vi "CreateSensorSession.vi"(8 "error in (no error)":errorcluster, 11 "SiemensDigitalEnergyMeter in":refnum<class "SiemensDigitalEnergyMeter.lvclass">) -> (0 "error out":errorcluster, 3 "SiemensDigitalEnergyMeter out":refnum<class "SiemensDigitalEnergyMeter.lvclass">)   [LabVIEW 2018, in "SensorPlugins.lvlib" / "SiemensDigitalEnergyMeter.lvclass"]
doc: "This VI opens a communication link between the application and the Siemens Digital Energy Meter using an IP address and a port number."
uses:
  SiemensDigitalEnergyMeter.lvclass
  <vilib>/NI/Modbus Library/API/Wrapper/Create Serial Master.vi
  <vilib>/NI/Modbus Library/API/Wrapper/Create TCP Master.vi
  <vilib>/NI/Modbus Library/API/Master/Modbus Master.lvclass
  <vilib>/NI/Modbus Library/API/Wrapper/API Main.lvlib
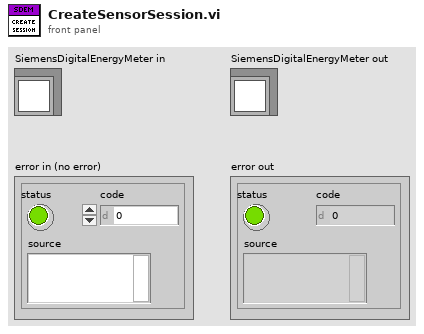
[diagram p1: front panel]
types:
  T1 = typedef "SensorPlugins.lvlib/SiemensDigitalEnergyMeter.lvclass/SiemensDigitalEnergyMeterControls.ctl" = cluster{"Measurement(s)":u16[], "Configuration Commands":string, "Use Measurement Commands Text Box?":bool, "Measurement Commands":string, "Connected?":bool, "Serial Number":string, "IP Address":string, "Port (502)":u16, "Unit ID":u8, "Serial Type":enum16{"RTU", "ASCII"}, "Using TCP?":bool, "VISA Resource Name":string}[]
  T2 = typedef "SensorPlugins.lvlib/SiemensDigitalEnergyMeter.lvclass/CommunicationControls.ctl" = refnum<class "Modbus Master.lvclass">[]
  T3 = cluster{"Measurement(s)":u16[], "Configuration Commands":string, "Use Measurement Commands Text Box?":bool, "Measurement Commands":string, "Connected?":bool, "Serial Number":string, "IP Address":string, "Port (502)":u16, "Unit ID":u8, "Serial Type":enum16{"RTU", "ASCII"}, "Using TCP?":bool, "VISA Resource Name":string}
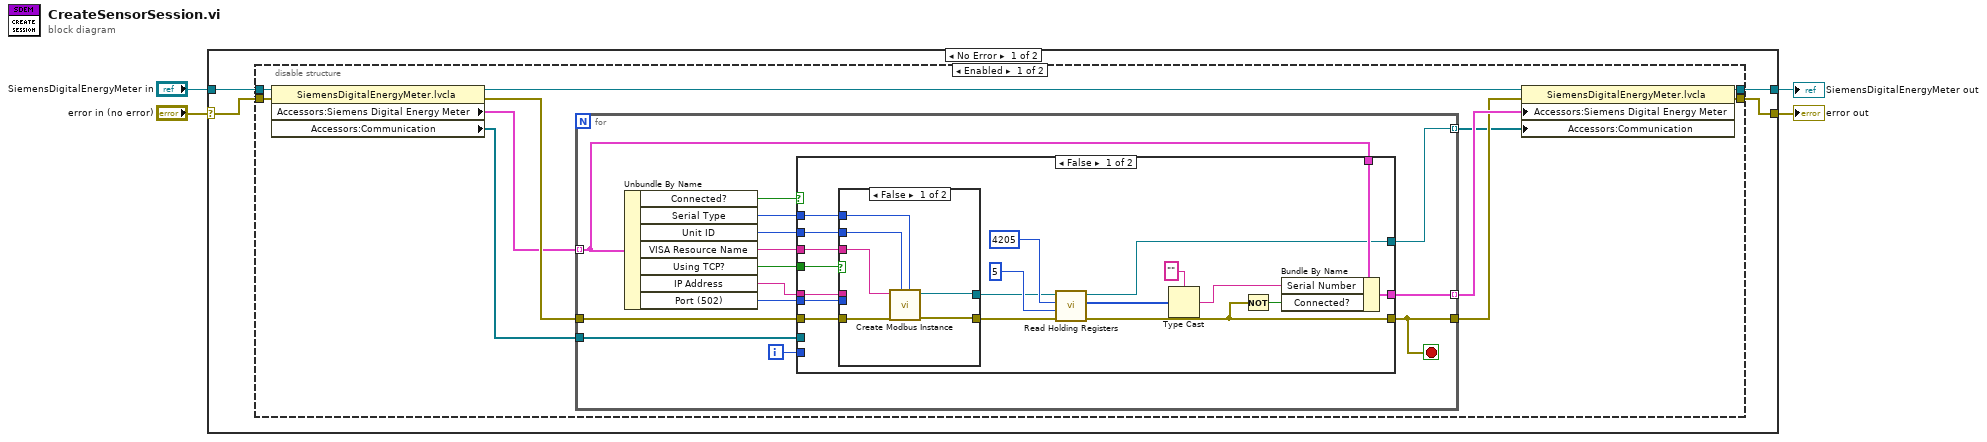
[diagram p0: block diagram]
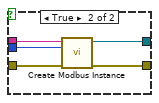
[diagram p2: hidden frame]
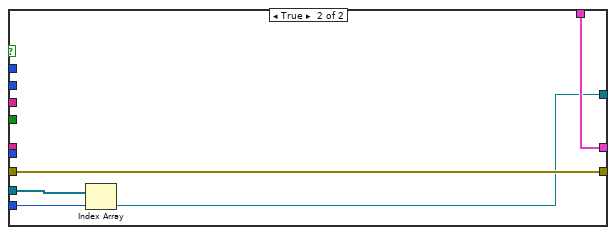
[diagram p3: hidden frame]
diagram:
  n1 = case shown="No Error" "error in (no error)" {
    selector: "error in (no error)" -> [w7 w71]
    tunnel: "SiemensDigitalEnergyMeter in" -> [w8 w72]
    tunnel: [w6 w72] -> w2
    tunnel: [w5 w71] -> w1
    frame No Error {
      n2 = disable-structure shown="Enabled" {
        disable-tunnel: w8 -> [w19 w70]
        disable-tunnel: w7 -> [w18 w69]
        disable-tunnel: [w15 w70] -> w6
        disable-tunnel: [w11 w69] -> w5
        frame Enabled {
          n3 = property class="SiemensDigitalEnergyMeter.lvcla"(reference=w19, error in=w18) -> (reference out=w14:refnum<class "SiemensDigitalEnergyMeter.lvclass">, error out=w17:errorcluster, "Accessors:Siemens Digital Energy Meter"=w16:T1, "Accessors:Communication"=w9:T2)
          n4 = for {
            tunnel: w17 -> [w31]
            tunnel: [w28] -> w12
            tunnel: w16 -> [w33] mode=indexing
            tunnel: [w32] -> w13 mode=indexing
            tunnel: [w27] -> w10 mode=indexing
            tunnel: w9 -> [w20]
            i -> [w21]
            stop <- w28 stop-if-true
            n5 = Unbundle By Name(w33) -> ("Connected?"=w22:bool, "Serial Type"=w23:enum16{"RTU", "ASCII"}, "Unit ID"=w24:u8, "VISA Resource Name"=w25:string, "Using TCP?"=w26:bool, "IP Address"=w30:string, "Port (502)"=w29:u16)
            n6 = case shown="False" w22 {
              tunnel: w33 -> [w52 w68]
              tunnel: [w51 w68] -> w32
              tunnel: w31 -> [w47 w67]
              tunnel: w30 -> [w46 _]
              tunnel: w29 -> [w45 _]
              tunnel: [w44 w67] -> w28
              tunnel: [w38 w64] -> w27
              tunnel: w26 -> [w37 _]
              tunnel: w25 -> [w36 _]
              tunnel: w24 -> [w35 _]
              tunnel: w23 -> [w34 _]
              tunnel: w21 -> [_ w66]
              tunnel: w20 -> [_ w65]
              frame False {
                n7 = case shown="False" w37 {
                  tunnel: w47 -> [w58 w63]
                  tunnel: w46 -> [_ w62]
                  tunnel: w45 -> [_ w61]
                  tunnel: [w57 w60] -> w43
                  tunnel: [w56 w59] -> w40
                  tunnel: w36 -> [w55 _]
                  tunnel: w35 -> [w54 _]
                  tunnel: w34 -> [w53 _]
                  frame False {
                    n8 = call-poly <vilib>:"Create Modbus Instance.vi"("serial type"=w53, "unit ID"=w54, "error in"=w58, "VISA resource name"=w55) -> ("error out"=w57:errorcluster, "serial master instance"=w56:refnum<class "Modbus Master.lvclass">)  [unwired: 6 in]
                  }
                  frame True {
                    n9 = call-poly <vilib>:"Create Modbus Instance.vi"("error in"=w63, "port (502)"=w61, "address"=w62) -> ("error out"=w60:errorcluster, "TCP master instance"=w59:refnum<class "Modbus Master.lvclass">)  [unwired: 7 in]
                  }
                }
                n10 = call-dynamic "Read Holding Registers.vi"("error in"=w43, "number of inputs"=u16 5 ("number of holding registers"), "starting address"=u16 4205, "Modbus master in"=w40) -> ("error out"=w44:errorcluster, "register values"=w39:u16[], "Modbus master out"=w38:refnum<class "Modbus Master.lvclass">)  [unwired: 5 in]
                n11 = Type Cast(type="", x=w39) -> (*(type *) &x=w48:string)
                n12 = Not(x=w44) -> (.not. x?=w50:bool)
                n13 = Bundle By Name(cluster=w52, "Serial Number"=w48, "Connected?"=w50) -> (w51:T3)
              }
              frame True {
                n14 = Index Array(array=w65, index=w66) -> (element=w64:refnum<class "Modbus Master.lvclass">)
              }
            }
          }
          n15 = property class="SiemensDigitalEnergyMeter.lvcla"(reference=w14, error in=w12, "Accessors:Siemens Digital Energy Meter"=w13, "Accessors:Communication"=w10) -> (reference out=w15:refnum<class "SiemensDigitalEnergyMeter.lvclass">, error out=w11:errorcluster)
        }
        frame Disabled {
        }
      }
    }
    frame Error {
    }
  }
  "error out" <- w1
  "SiemensDigitalEnergyMeter out" <- w2
